vi "Test Get Pin Status Comm.vi"(8 "error in (no error)":errorcluster, 11 "TestCase in":refnum<class "Test Get Pin Status.lvclass">) -> (0 "error out":errorcluster, 3 "TestCase out":refnum<class "Test Get Pin Status.lvclass">)   [LabVIEW 2020, in "Test Get Pin Status.lvclass"]
uses:
  Test Get Pin Status.lvclass
  Implementations/Simulado/Simulado.lvclass
  <vilib>/addons/_JKI Toolkits/VI Tester/TestCase.llb/TestCase.lvclass
  C:/Program Files (x86)/National Instruments/LabVIEW 2020/vi.lib/addons/_JKI Toolkits/VI Tester/TestCase.llb/TestCase.lvclass
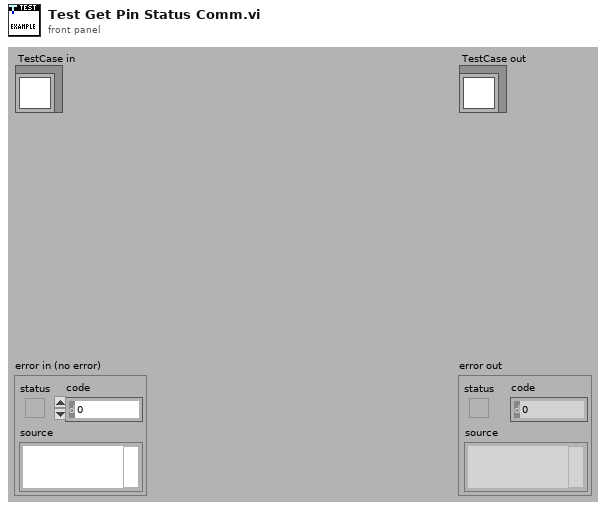
[diagram p1: front panel]
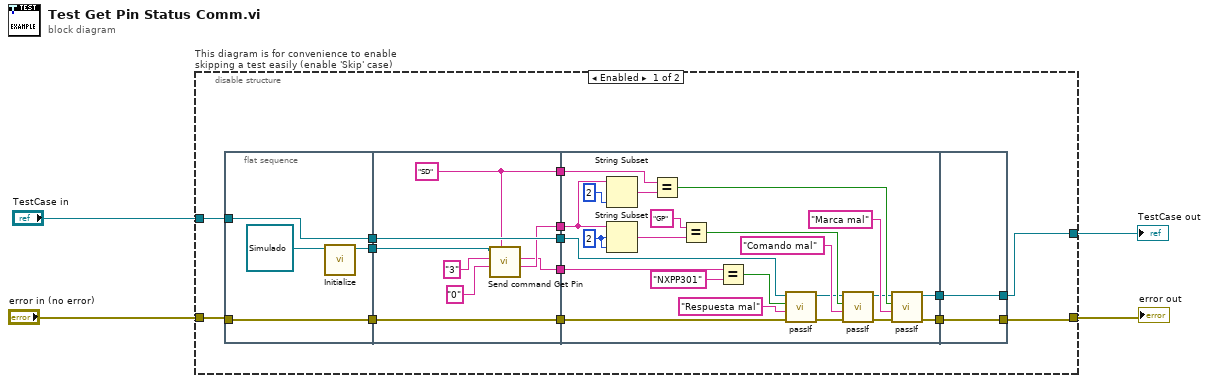
[diagram p0: block diagram]
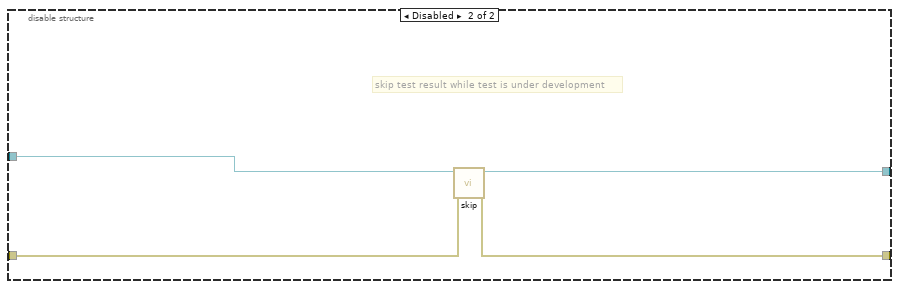
[diagram p2: hidden frame]
diagram:
  n1 = disable-structure "This diagram is for convenience to enable skipping a test easily (enable 'Skip' case)" shown="Enabled" {
    disable-tunnel: "TestCase in" -> [w6 w59]
    disable-tunnel: [w8 w57] -> w1
    disable-tunnel: [w7 w58] -> w3
    disable-tunnel: "error in (no error)" -> [w5 w56]
    frame Enabled {
      n2 = flat-sequence {
        tunnel: w6 -> [w22]
        tunnel: [w22] -> w18
        tunnel: w5 -> [w21]
        tunnel: [w21] -> w17
        tunnel: [w19] -> w16
        tunnel: [w30] -> w15
        tunnel: w18 -> [w30]
        tunnel: [w29] -> w14
        tunnel: w17 -> [w29]
        tunnel: w16 -> [w28]
        tunnel: [w27] -> w13
        tunnel: [w26] -> w12
        tunnel: [w23] -> w11
        tunnel: [w50] -> w10
        tunnel: w15 -> [w36]
        tunnel: [w49] -> w9
        tunnel: w14 -> [w34]
        tunnel: w13 -> [w39]
        tunnel: w12 -> [w38]
        tunnel: w11 -> [w51]
        tunnel: [w55] -> w8
        tunnel: w10 -> [w55]
        tunnel: [w54] -> w7
        tunnel: w9 -> [w54]
        frame #0 {
          n3 = call-dynamic "Initialize.vi"("object in"=refnum<class "Simulado.lvclass"> refnum ("Simulado.lvclass")) -> ("object out"=w19:refnum<class "Simulado.lvclass">)  [unwired: 9 in, 1 out]
        }
        frame #1 {
          w23 = "SD" ("Marca")
          n4 = call-dynamic "Send command Get Pin.vi"("Marca"=w23, "Pin"="0", "Puerto"="3", "Simulado in"=w28) -> ("Command"=w27:string, "Expected response"=w26:string)  [unwired: 4 in, 2 out]
        }
        frame #2 {
          w46 = 2 ("length (rest)")
          n5 = String Subset(string=w39, length (rest)=2 ("length (rest)")) -> (substring=w52:string)  [unwired: 1 in]
          n6 = String Subset(string=w39, offset (0)=w46, length (rest)=w46) -> (substring=w45:string)
          n7 = Equal?(x=w51, y=w52) -> (x = y?=w48:bool)
          n8 = Equal?(x="GP", y=w45) -> (x = y?=w41:bool)
          n9 = Equal?(x=w38, y="NXPP301") -> (x = y?=w32:bool)
          n10 = call-dynamic "passIf.vi"("error in (no error)"=w34, "message (\"\")"="Respuesta mal" ("message (\"\")"), "pass"=w32, "TestCase in"=w36) -> ("error out"=w33:errorcluster, "TestCase out"=w35:refnum<class "Test Get Pin Status.lvclass">)  [unwired: 6 in]
          n11 = call-dynamic "passIf.vi"("error in (no error)"=w33, "message (\"\")"="Comando mal" ("message (\"\")"), "pass"=w41, "TestCase in"=w35) -> ("error out"=w42:errorcluster, "TestCase out"=w43:refnum<class "Test Get Pin Status.lvclass">)  [unwired: 6 in]
          n12 = call-dynamic "passIf.vi"("error in (no error)"=w42, "message (\"\")"="Marca mal" ("message (\"\")"), "pass"=w48, "TestCase in"=w43) -> ("error out"=w49:errorcluster, "TestCase out"=w50:refnum<class "Test Get Pin Status.lvclass">)  [unwired: 6 in]
        }
        frame #3 {
        }
      }
    }
    frame Disabled {
      # "skip test result while test is under development"
      n13 = call <vilib>:"skip.vi"("error in (no error)"=w56, "TestCase in"=w59) -> ("error out"=w58:errorcluster, "TestCase out"=w57:refnum<class "Test Get Pin Status.lvclass">)  [unwired: 8 in]
    }
  }
  "error out" <- w3
  "TestCase out" <- w1
